vi "Point At.vi"(9 "Up":T1, 10 "Target":T1, 11 "Position":T1) -> (3 "Point At Matrix":sgl[][](array[numeric]))   [LabVIEW 2022 SP3, in "3D.lvlib"]
uses:
  3D.lvlib
  Vector 3D.ctl
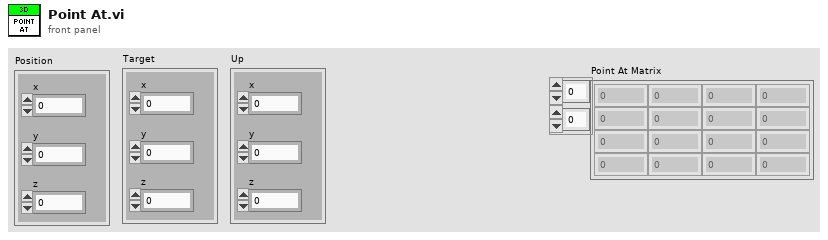
[diagram p1: front panel]
types:
  T1 = typedef "3D.lvlib/Vector 3D.ctl" = cluster{"x":sgl, "y":sgl, "z":sgl}
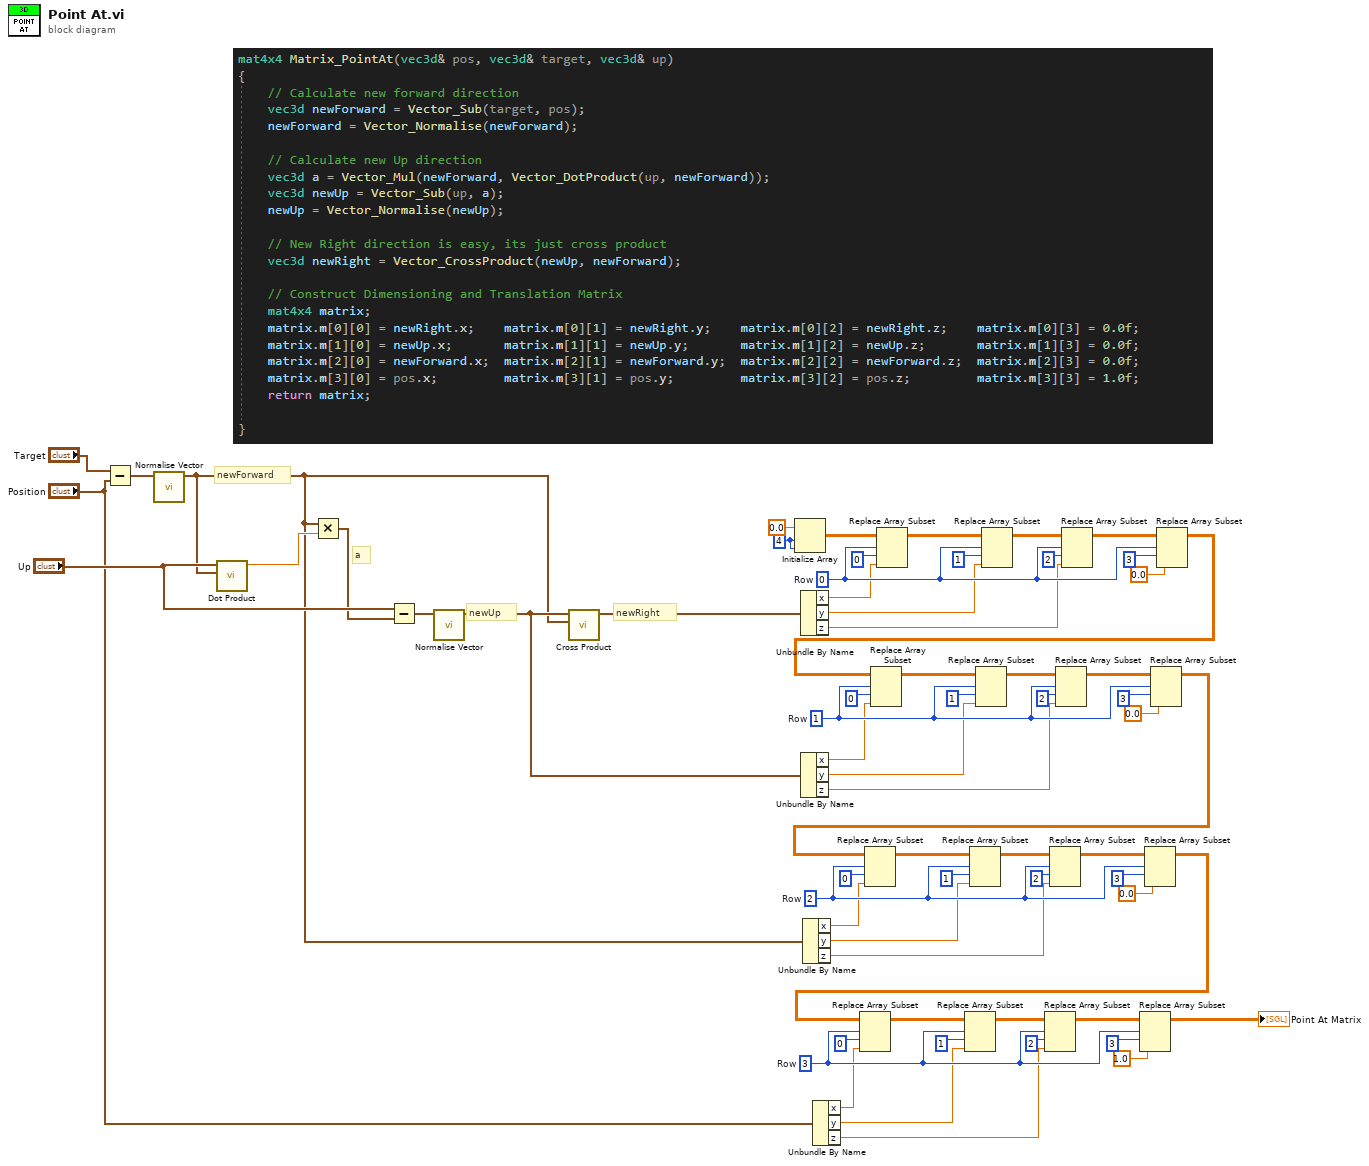
[diagram p0: block diagram]
diagram:
  w30 = 3  # Row
  w32 = 2  # Row
  w48 = 1  # Row
  w49 = 0  # Row
  w58 = 4 ("dimension size")
  # "a"
  # "newUp"
  # "newForward"
  # "newRight"
  n1 = Subtract(x="Target", y="Position") -> (x-y=w64:T1)
  n2 = call "Normalise Vector.vi"("Vector 3D"=w64) -> ("Vector 3D Normalised"=w10:T1)  [unwired: 10 in]
  n3 = call "Dot Product.vi"("Vector B"=w10, "Vector A"="Up") -> ("Dot Product"=w63:sgl)  [unwired: 9 in]
  n4 = Multiply(x=w10, y=w63) -> (x*y=w61:T1)
  n5 = Subtract(x="Up", y=w61) -> (x-y=w60:T1)
  n6 = call "Normalise Vector.vi"("Vector 3D"=w60) -> ("Vector 3D Normalised"=w15:T1)  [unwired: 10 in]
  n7 = call "Cross Product.vi"("Vector B"=w10, "Vector A"=w15) -> ("Cross Product"=w20:T1)  [unwired: 9 in]
  n8 = Initialize Array(sgl 0.0 ("element"), w58, w58) -> (w57:sgl[][])
  n9 = Unbundle By Name(w20) -> ("x"=w19:sgl, "y"=w18:sgl, "z"=w17:sgl)
  n10 = Unbundle By Name(w15) -> ("x"=w14:sgl, "y"=w13:sgl, "z"=w12:sgl)
  n11 = Unbundle By Name(w10) -> ("x"=w9:sgl, "y"=w8:sgl, "z"=w7:sgl)
  n12 = Unbundle By Name("Position") -> ("x"=w4:sgl, "y"=w3:sgl, "z"=w2:sgl)
  n13 = Replace Array Subset(array=w57, new element=w19, index (row)=w49, index (col)=0 ("index (row)")) -> (w54:sgl[][])
  n14 = Replace Array Subset(array=w54, new element=w18, index (row)=w49, index (col)=1 ("index (row)")) -> (w52:sgl[][])
  n15 = Replace Array Subset(array=w52, new element=w17, index (row)=w49, index (col)=2 ("index (row)")) -> (w50:sgl[][])
  n16 = Replace Array Subset(array=w50, new element=sgl 0.0 ("new element/subarray"), index (row)=w49, index (col)=3 ("index (row)")) -> (w40:sgl[][])
  n17 = Replace Array Subset(array=w40, new element=w14, index (row)=w48, index (col)=0 ("index (row)")) -> (w43:sgl[][])
  n18 = Replace Array Subset(array=w43, new element=w13, index (row)=w48, index (col)=1 ("index (row)")) -> (w45:sgl[][])
  n19 = Replace Array Subset(array=w45, new element=w12, index (row)=w48, index (col)=2 ("index (row)")) -> (w47:sgl[][])
  n20 = Replace Array Subset(array=w47, new element=sgl 0.0 ("new element/subarray"), index (row)=w48, index (col)=3 ("index (row)")) -> (w31:sgl[][])
  n21 = Replace Array Subset(array=w31, new element=w9, index (row)=w32, index (col)=0 ("index (row)")) -> (w37:sgl[][])
  n22 = Replace Array Subset(array=w37, new element=w8, index (row)=w32, index (col)=1 ("index (row)")) -> (w35:sgl[][])
  n23 = Replace Array Subset(array=w35, new element=w7, index (row)=w32, index (col)=2 ("index (row)")) -> (w33:sgl[][])
  n24 = Replace Array Subset(array=w33, new element=sgl 0.0 ("new element/subarray"), index (row)=w32, index (col)=3 ("index (row)")) -> (w22:sgl[][])
  n25 = Replace Array Subset(array=w22, new element=w4, index (row)=w30, index (col)=0 ("index (row)")) -> (w25:sgl[][])
  n26 = Replace Array Subset(array=w25, new element=w3, index (row)=w30, index (col)=1 ("index (row)")) -> (w27:sgl[][])
  n27 = Replace Array Subset(array=w27, new element=w2, index (row)=w30, index (col)=2 ("index (row)")) -> (w29:sgl[][])
  n28 = Replace Array Subset(array=w29, new element=sgl 1.0 ("new element/subarray"), index (row)=w30, index (col)=3 ("index (row)")) -> (→"Point At Matrix":sgl[][])
